vi "Enable Disable.vi"(8 "error in":errorcluster, 11 "Node Ptr":u64 format="%.0x") -> (0 "error out":errorcluster)   [LabVIEW 2027, in "Embedded Data Logger System Explorer.lvlib"]
uses:
  Embedded Data Logger System Explorer.lvlib
  Scripting/Embedded Data Logger Scripting.lvlib
panel:
  in  "Tag":string
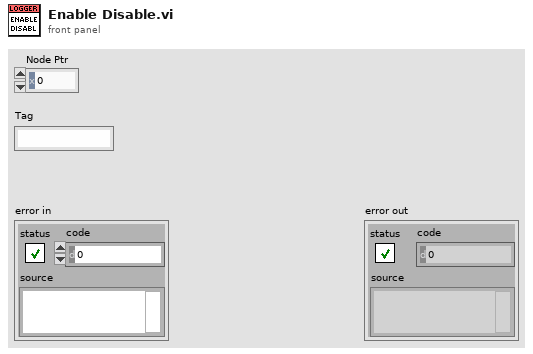
[diagram p1: front panel]
types:
  T1 = typedef "Custom Device API.lvlib/Custom Device Item Ref.ctl" = u64
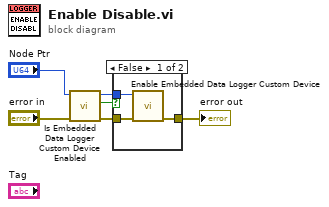
[diagram p0: block diagram]
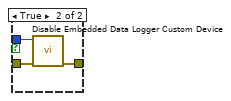
[diagram p2: hidden frame]
diagram:
  n1 = call "Is Embedded Data Logger Custom Device Enabled.vi"("error in"="error in", "embedded data logger in"="Node Ptr") -> ("error out"=w2:errorcluster, "enabled"=w6:bool, "embedded data logger out"=w3:T1)  [unwired: 7 in]
  n2 = case shown="False" w6 {
    tunnel: [w9 w10] -> w1
    tunnel: w3 -> [w8 w11]
    tunnel: w2 -> [w7 w12]
    frame False {
      n3 = call "Enable Embedded Data Logger Custom Device.vi"("error in"=w7, "embedded data logger in"=w8) -> ("error out"=w9:errorcluster)  [unwired: 8 in, 1 out]
    }
    frame True {
      n4 = call "Disable Embedded Data Logger Custom Device.vi"("error in"=w12, "embedded data logger in"=w11) -> ("error out"=w10:errorcluster)  [unwired: 8 in, 1 out]
    }
  }
  "error out" <- w1
